vi "waveTest.vi"() -> ()   [LabVIEW 2018]
uses:
  <vilib>/measure/NI_MABase.lvlib
panel:
  in  "png?":bool=TRUE
  out "standard output":string
  out "output png":picture
  in  "amplitude":dbl=21.0 format="%0.2p"
  in  "frequency":dbl=3.0 format="%0.2p"
  in  "signal type":T1(ring)=enum."Triangle Wave"
  in  "add noise":bool=TRUE
  in  "number of points":dbl(slide)=44.4776119402985 scale=10.0..1000.0
  out "LaTeX output":string
  out "Waveform Graph":waveform(dbl)[](graph)=[{"t0"=timestamp(0 s since 1904-01-01), "dt"=0.02248322147651007, "Y"=[-1.546477433388504, 4.661984807620563, 7.8278201832138725, 11.001512342104604, 15.015062026967165, 15.512826662722626, 15.574358460996109, 13.290410667596724, 11.99348612908547, 8.588629763986237, 5.067512693167407, 1.258457503857374, -2.8810456117563374, -6.925805192568073, -10.545354256767709, -14.932883970541788, -13.577918727803066, -14.589587562163713, -11.46193309140618, -12.290200153543955, -9.437814005181771, -4.8264367558785795, -1.2386574847111085, 3.051340081786596, 6.950914289149695, 9.981049349063406, 12.35566247672647, 15.294188005780697, 14.350046666102049, 14.978056870639572, 13.443684958705374, 9.524808574601101, 5.281310569613, 0.09035510962493731, -3.3367521947681373, -5.625031359450402, -10.134935689127893, -12.522309407667565, -13.59685597158344, -14.168685301718552, -14.20184362459651, -12.77561767255461, -10.526530375259396, -7.10442228803309]}, {"t0"=timestamp(0 s since 1904-01-01), "dt"=0.001, "Y"=array[1000 elements]}]
  in  "Amplitude":dbl(slide)=15.016835016835017 scale=0.0..20.0
  # "first signal"
  # "second signal"
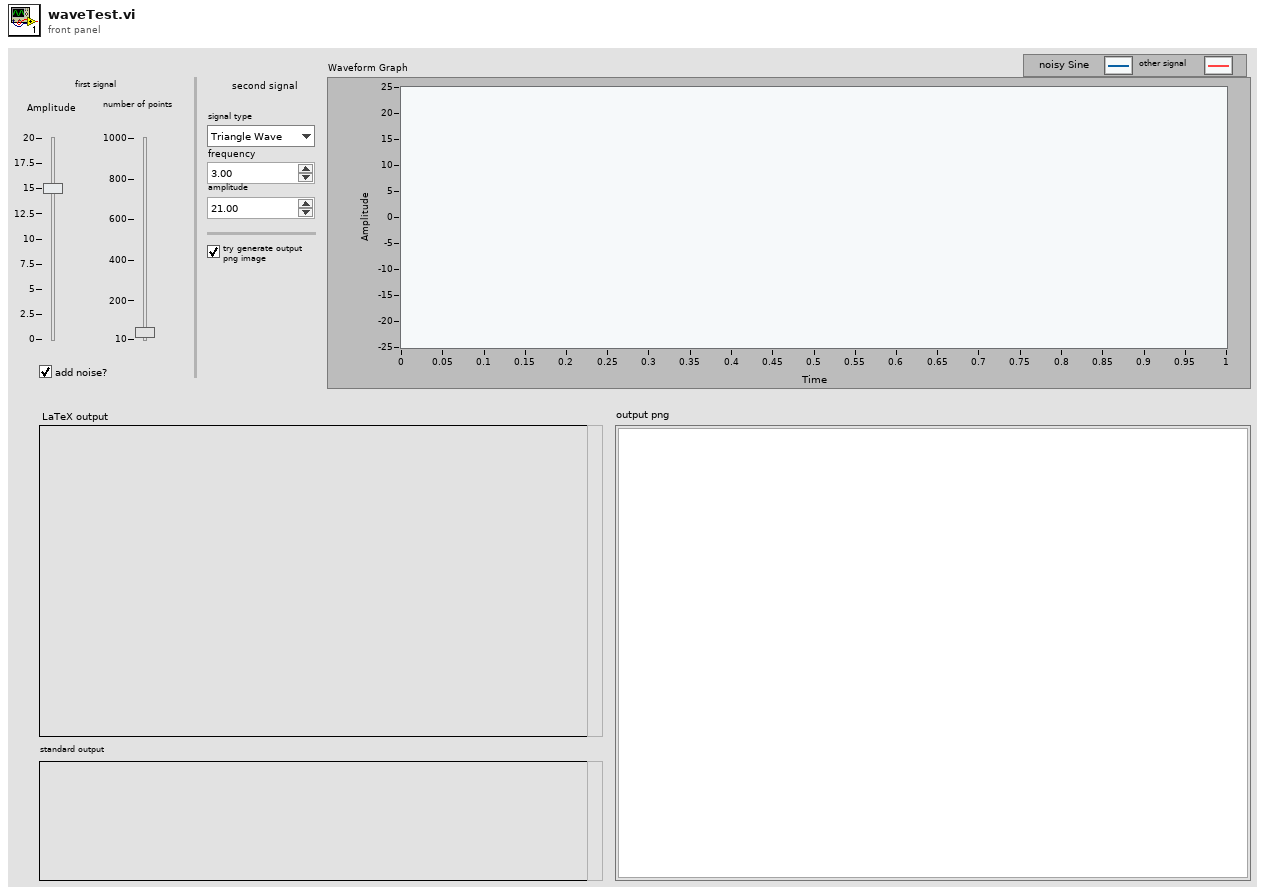
[diagram p1: front panel]
types:
  T1 = enum16{"Sine Wave", "Triangle Wave", "Square Wave", "Sawtooth Wave"}
  T2 = typedef "LVBoundsTypeDef.ctl" = cluster{"Width":u32, "Height":u32}
  T3 = typedef "imagedata.ctl" = cluster{"image type":i32, "image depth":i32, "image":u8[], "mask":u8[], "colors":u32[], "Rectangle":cluster{"left":i16, "top":i16, "right":i16, "bottom":i16}}
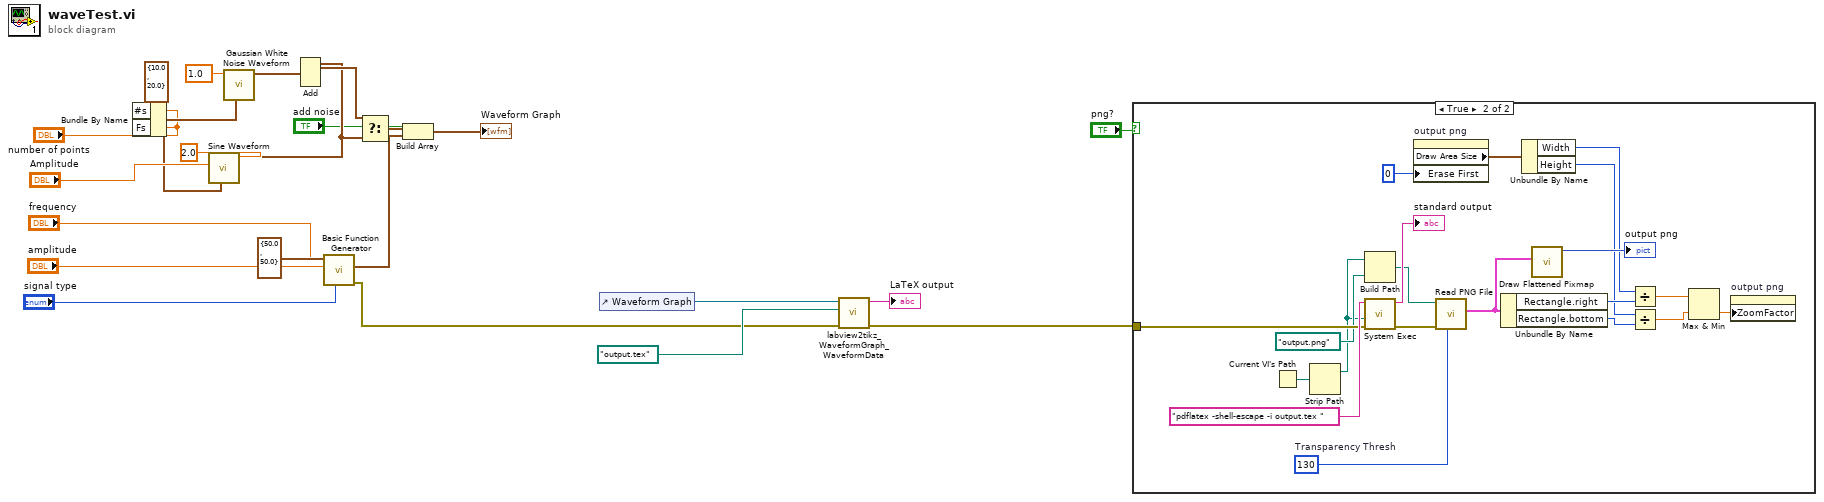
[diagram p0: block diagram]
diagram:
  n1 = Bundle By Name(cluster=cluster{"Fs":dbl, "#s":dbl} {"Fs"=10.0, "#s"=20.0} ("sampling info"), "#s"="number of points", "Fs"="number of points") -> (w15:cluster{"Fs":dbl, "#s":dbl})
  n2 = call <vilib>:"Sine Waveform.vi"("sampling info"=w15, "amplitude"="Amplitude", "frequency"=2.0 ("Frequency")) -> ("signal out"=w12:waveform(dbl))  [unwired: 7 in, 1 out]
  n3 = call <vilib>:"Gaussian White Noise Waveform.vi"("sampling info"=w15, "standard deviation"=1.0) -> ("signal out"=w23:waveform(dbl))  [unwired: 8 in, 1 out]
  n4 = Add(1:w23, 2:w12) -> (0:w13:waveform(dbl))  [unwired: 1 in, 1 out]
  n5 = call <vilib>:"Basic Function Generator.vi"("sampling info"=cluster{"Fs":dbl, "#s":dbl} {"Fs"=50.0, "#s"=50.0}, "signal type"="signal type", "amplitude"="amplitude", "frequency"="frequency") -> ("error out"=w2:errorcluster, "signal out"=w9:waveform(dbl))  [unwired: 5 in, 1 out]
  n6 = Select(t=w13, s="add noise", f=w12) -> (s? t:f=w11:waveform(dbl))
  n7 = Build Array(w11, w9) -> (→"Waveform Graph":waveform(dbl)[])
  n8 = control-ref of="Waveform Graph"() -> (w1:refnum<vi>)
  n9 = call "labview2tikz_WaveformGraph_WaveformData.vi"("error in (no error)"=w2, "file (use dialog)"=path "output.tex", "WaveformGraph in"=w1) -> ("error out"=w4:errorcluster, "result string"=→"LaTeX output":string)  [unwired: 7 in]
  n10 = case shown="True" "png?" {
    tunnel: w4 -> [_ w42]
    frame False {
    }
    frame True {
      w34 = u8 130  # Transparency Thresh
      n11 = Current VI's Path() -> (path=w38:path)
      n12 = Strip Path(path=w38) -> (stripped path=w35:path)  [unwired: 1 out]
      n13 = Build Path(base path=w35, name or relative path=path "output.png" ("file (use dialog)")) -> (appended path=w37:path)
      n14 = call <vilib>:"System Exec.vi"("error in (no error)"=w42, "working directory"=w35, "command line"="pdflatex -shell-escape -i output.tex ") -> ("error out"=w40:errorcluster, "standard output"=→"standard output":string)  [unwired: 5 in, 2 out]
      n15 = property on="output png" class="Pict"("Erase First"=u8 0) -> ("Draw Area Size"=w32:T2)  [unwired: 2 in, 2 out]
      n16 = call <vilib>:"Read PNG File.vi"("Transparency Thresh"=w34, "error in (no error)"=w40, "path to PNG file"=w37) -> ("image data"=w24:T3)  [unwired: 6 in, 2 out]
      n17 = Unbundle By Name(w24) -> ("Rectangle.right"=w30:i16, "Rectangle.bottom"=w28:i16)
      n18 = Unbundle By Name(w32) -> ("Width"=w31:u32, "Height"=w29:u32)
      n19 = call <vilib>:"Draw Flattened Pixmap.vi"("image data"=w24) -> ("new picture"=→"output png":picture)  [unwired: 8 in]
      n20 = Divide(x=w31, y=w30) -> (x/y=w27:dbl)
      n21 = Divide(x=w29, y=w28) -> (x/y=w26:dbl)
      n22 = Max & Min(x=w27, y=w26) -> (min(x,y)=w25:dbl)  [unwired: 1 out]
      n23 = property on="output png" class="Pict"("ZoomFactor"=w25) -> ()  [unwired: 2 in, 2 out]
    }
  }
